vi "Get dt.vi"(1 "options":T1={"sp low"=0.0, "sp high"=100.0, "out low"=-100.0, "out high"=100.0, "hold (F)"=FALSE, "auto (T)"=TRUE, "pro. band (F)"=FALSE, "reverse acting (T)"=TRUE, "beta"=1.0, "linearity"=1.0, "dt (s)"=-1.0} {"dt (s)" format="%.2f"; "linearity" min=0.0 max=1.0 format="%.2f"; "sp low" format="%.2f"; "sp high" format="%.2f"; "out low" format="%.2f"; "out high" format="%.2f"; "beta" min=0.0 max=1.0 format="%.2f"}) -> (0 "dt (min.)":dbl format="%.2f")   [LabVIEW 2012]
doc: "This VI calculates the time interval between calls to the PID function when the optional input dt (s) is -1."
panel:
  # "SP & PV range:"
  # "Output range:"
  # "-1: default,using\nsystem clock"
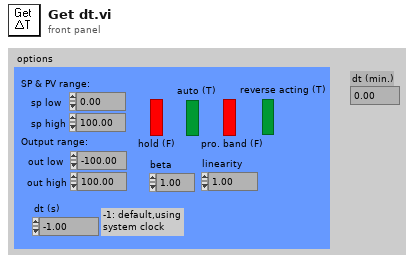
[diagram p1: front panel]
types:
  T1 = cluster{"sp low":dbl, "sp high":dbl, "out low":dbl, "out high":dbl, "hold (F)":bool, "auto (T)":bool, "pro. band (F)":bool, "reverse acting (T)":bool, "beta":dbl, "linearity":dbl, "dt (s)":dbl}
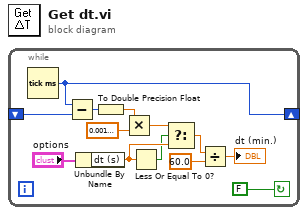
[diagram p0: block diagram]
diagram:
  n1 = while {
    shift-left: _ -> [w3]
    shift-right: [w4] -> _
    stop <- FALSE continue-if-true
    n2 = Tick Count (ms)() -> (millisecond timer value=w4:u32)
    n3 = Subtract(x=w4, y=w3) -> (x-y=w10:u32)
    n4 = Unbundle By Name("options") -> ("dt (s)"=w13:dbl)
    n5 = To Double Precision Float(number=w10) -> (double precision float=w9:dbl)
    n6 = Multiply(x=w9, y=0.0010000000474974513) -> (x*y=w7:dbl)
    n7 = Less Or Equal To 0?(x=w13) -> (x <= 0?=w6:bool)
    n8 = Select(t=w7, s=w6, f=w13) -> (s? t:f=w8:dbl)
    n9 = Divide(x=w8, y=60.0) -> (x/y=→"dt (min.)":dbl)
  }
